vi "Host_HoppingScan(XZ_FPGAWithin).vi"() -> ()   [LabVIEW 2014]
uses:
  <vilib>/userdefined/High Color/nirio_resource_hc.ctl
  <vilib>/Native 3D Graph/xcontrol/3DPC_SurfacePlot.xctl
  <vilib>/Instr/_visa.llb/VISA Configure Serial Port (Instr).vi
  <vilib>/FPGAPlugInAG/PCIe-7851R/niLvFpga_Open_PCIe-7851R.vi
  <vilib>/rvi/interface/common/dynamic/niFpgaDynamicAddResources.vi
  <vilib>/Utility/error.llb/Error Cluster From Error Code.vi
  <vilib>/rvi/errors/niLvFpgaAdjustHostInterfaceError.vi
  <vilib>/FPGAPlugInAG/Dynamic/niLvFpga_Close_Dynamic.vi
  <vilib>/rvi/interface/nirviOpenFPGA/nirviOpenFPGA.xnode
  FPGA Bitfiles/XZFPGAWithinHopp_FPGATarget_HoppingStep(Nonl_ZQj-tD8XJbo.lvbitx
  <vilib>/rvi/interface/nirviReadWriteControl/nirviReadWriteControl.xnode
  <vilib>/rvi/interface/nirviMethod/nirviMethod.xnode
  <vilib>/rvi/interface/nirviCloseFPGA/nirviCloseFPGA.xnode
  NiFpgaLv.dll
  <vilib>/rvi/interface/Simulation/niFpgaSimulationCallBeginRW.vi
  <vilib>/FPGAPlugInAG/Dynamic/niLvFpga_ReadFifo_Dynamic.vi
  <vilib>/rvi/errors/niLvFpgaMergeErrorWithErrorCode.vi
  <vilib>/FPGAPlugInAG/Dynamic/niLvFpga_StopFifo_Dynamic.vi
panel:
  out "XGetNum":u32
  in  "Relative?":bool
  in  "BottomSleep us":i32
  in  "UpperSleep us":i32
  out "SecElapsed s":dbl
  in  "UseCompensation":bool
  in  "Compensation / line":i32
  in  "RelativeWithdraw index":i32
  out "YPresPos":i32
  out "XBuffer":u32
  out "Waveform Chart":i32(graph)
  out "3D Graph":refnum<class "Base Datatype.lvclass">[](xcontrol)
  in  "stop":bool
  in  "ZOffset index":i32
  out "YPos?":dbl
  in  "YNum":i16
  in  "XNum":i16
  in  "YStepLen um":dbl format="%#_13g"
  in  "XStepMultiplier / 0.47nm":i16
  in  "XInitPos um":dbl format="%#_13g"
  in  "YInitPos um":dbl format="%#_13g"
  in  "PIXZ":T1
  out "ERR?":string
  in  "PIYDigital":refnum<visa-resource-name>
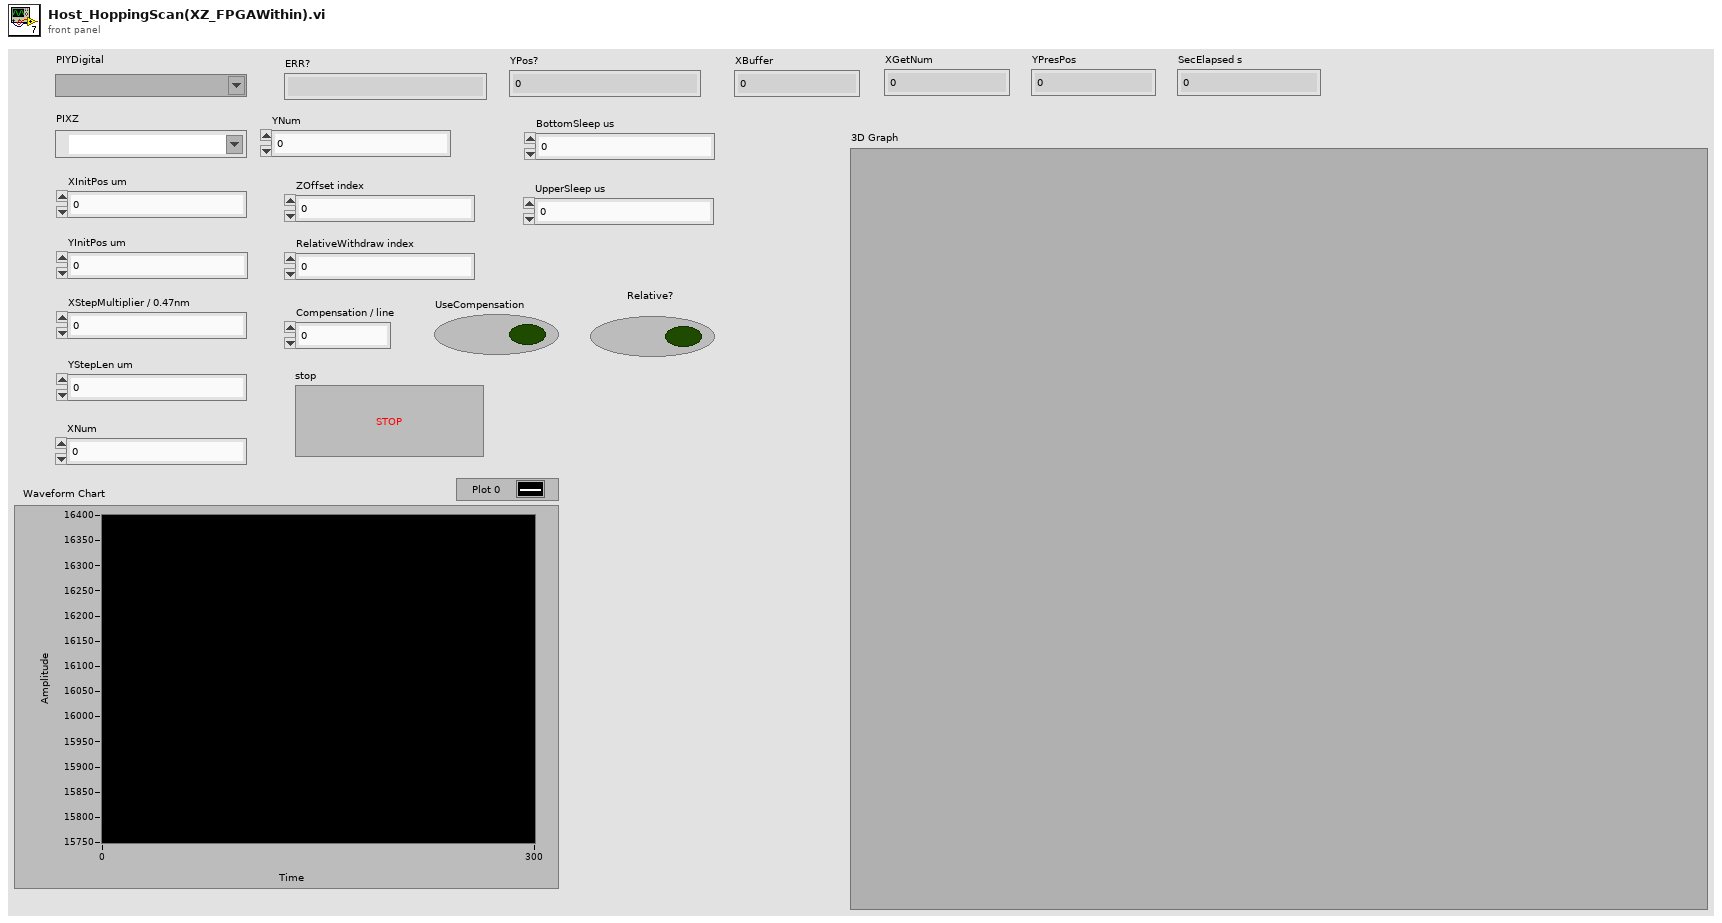
[diagram p1: front panel]
types:
  T1 = typedef "nirio_resource_hc.ctl" = tag
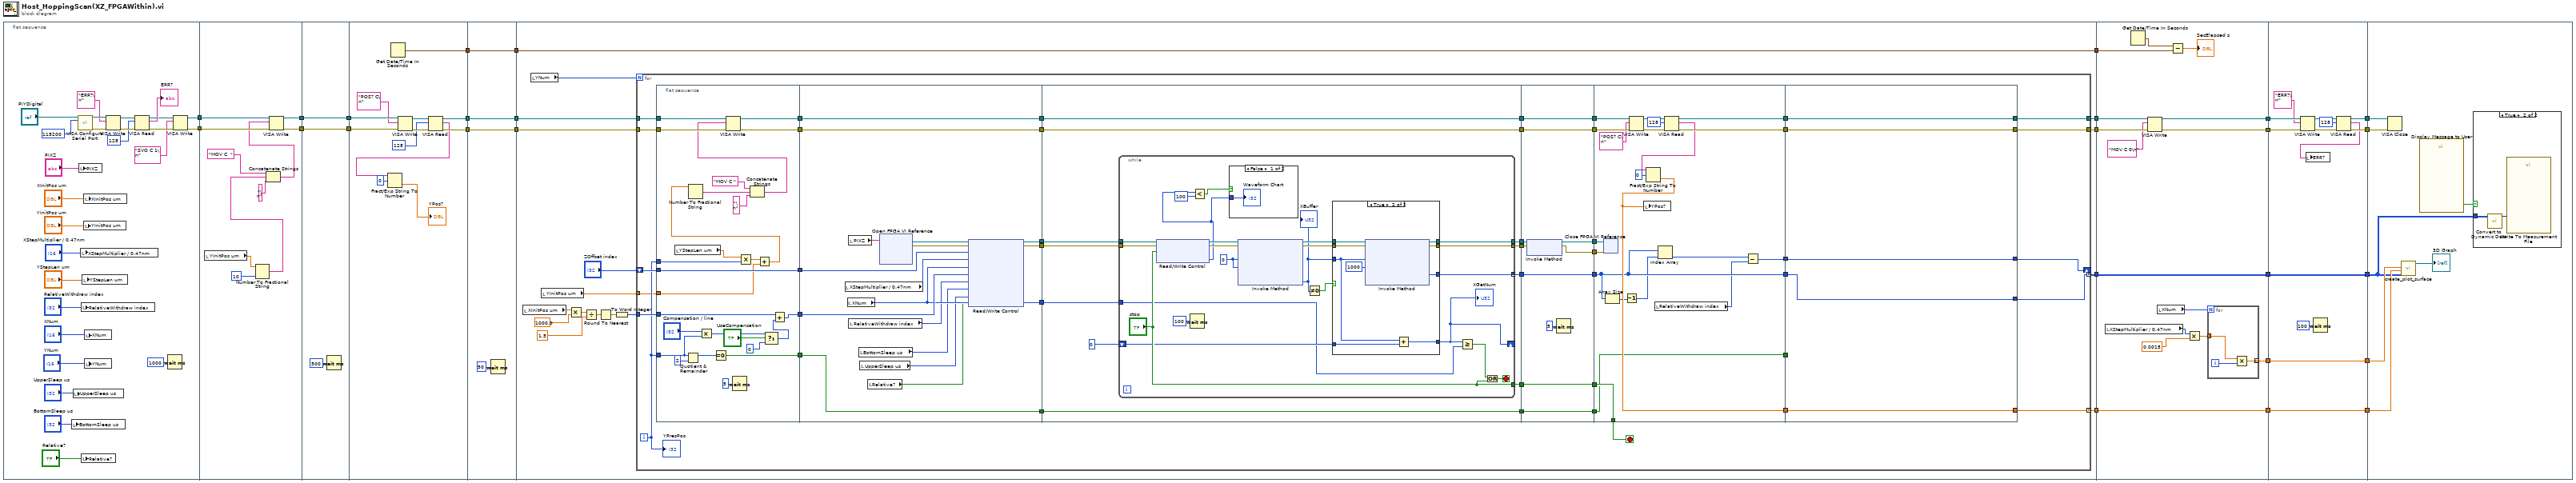
[diagram p0: block diagram]
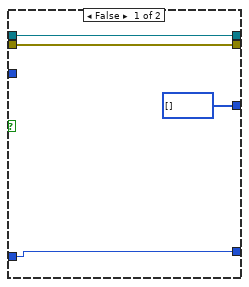
[diagram p3: hidden frame]
diagram:
  n1 = flat-sequence {
    tunnel: [w33] -> w27
    tunnel: [w32] -> w26
    tunnel: w27 -> [w63]
    tunnel: w26 -> [w62]
    tunnel: [w58] -> w25
    tunnel: [w57] -> w24
    tunnel: w25 -> [w65]
    tunnel: w24 -> [w64]
    tunnel: [w65] -> w23
    tunnel: [w64] -> w22
    tunnel: w23 -> [w78]
    tunnel: w22 -> [w77]
    tunnel: [w72] -> w21
    tunnel: [w71] -> w20
    tunnel: [w67] -> w2
    tunnel: w21 -> [w81]
    tunnel: w20 -> [w80]
    tunnel: [w81] -> w19
    tunnel: [w80] -> w18
    tunnel: [w79] -> w3
    tunnel: w2 -> [w79]
    tunnel: w19 -> [w98]
    tunnel: w18 -> [w97]
    tunnel: [w89] -> w17
    tunnel: [w88] -> w16
    tunnel: [w87] -> w11
    tunnel: [w86] -> w10
    tunnel: w3 -> [w83]
    tunnel: [w83] -> w1
    tunnel: w17 -> [w282]
    tunnel: w16 -> [w281]
    tunnel: [w279] -> w15
    tunnel: [w278] -> w14
    tunnel: w11 -> [w271]
    tunnel: w10 -> [w272]
    tunnel: [w273] -> w9
    tunnel: [w272] -> w6
    tunnel: [w271] -> w4
    tunnel: w1 -> [w270]
    tunnel: w15 -> [w298]
    tunnel: w14 -> [w297]
    tunnel: [w292] -> w13
    tunnel: [w291] -> w12
    tunnel: w9 -> [w288]
    tunnel: [w288] -> w8
    tunnel: [w287] -> w7
    tunnel: w6 -> [w287]
    tunnel: [w286] -> w5
    tunnel: w4 -> [w286]
    tunnel: w13 -> [w305]
    tunnel: w12 -> [w304]
    tunnel: w8 -> [w302]
    tunnel: w7 -> [w301]
    tunnel: w5 -> [w299]
    frame #0 {
      n2 = local write "BottomSleep us"("BottomSleep us") -> ()
      n3 = local write "UpperSleep us"("UpperSleep us") -> ()
      n4 = call-poly "VISA Configure Serial Port"("VISA resource name"="PIYDigital", "baud rate (9600)"=u32 115200) -> ("VISA resource name out"=w51:refnum<visa-resource-name>, "error out"=w50:errorcluster)  [unwired: 12 in]
      n5 = local write "PIXZ"("PIXZ") -> ()
      n6 = local write "XStepMultiplier / 0.47nm"("XStepMultiplier / 0.47nm") -> ()
      n7 = local write "RelativeWithdraw index"("RelativeWithdraw index") -> ()
      n8 = local write "Relative?"("Relative?") -> ()
      n9 = local write "YStepLen um"("YStepLen um") -> ()
      n10 = local write "YInitPos um"("YInitPos um") -> ()
      n11 = local write "XInitPos um"("XInitPos um") -> ()
      n12 = local write "XNum"("XNum") -> ()
      n13 = local write "YNum"("YNum") -> ()
      n14 = VISA Write(VISA resource name=w51, write buffer="ERR?\n", error in (no error)=w50) -> (VISA resource name out=w48:refnum<visa-resource-name>, error out=w47:errorcluster)  [unwired: 1 out]
      n15 = VISA Read(VISA resource name=w48, byte count=u32 128, error in (no error)=w47) -> (VISA resource name out=w35:refnum<visa-resource-name>, read buffer=→"ERR?":string, error out=w34:errorcluster)  [unwired: 1 out]
      n16 = Wait (ms)(milliseconds to wait=u32 1000) -> ()  [unwired: 1 out]
      n17 = VISA Write(VISA resource name=w35, write buffer="SVO C 1\n", error in (no error)=w34) -> (VISA resource name out=w33:refnum<visa-resource-name>, error out=w32:errorcluster)  [unwired: 1 out]
    }
    frame #1 {
      n18 = local read "YInitPos um"() -> (w56:dbl)
      n19 = Number To Fractional String(number=w56, precision (6)=i16 10) -> (F-format string=w54:string)  [unwired: 2 in]
      n20 = Concatenate Strings("MOV C  " ("write buffer"), w54, "\n" ("string")) -> (w59:string)
      n21 = VISA Write(VISA resource name=w63, write buffer=w59, error in (no error)=w62) -> (VISA resource name out=w58:refnum<visa-resource-name>, error out=w57:errorcluster)  [unwired: 1 out]
    }
    frame #2 {
      n22 = Wait (ms)(milliseconds to wait=u32 500) -> ()  [unwired: 1 out]
    }
    frame #3 {
      n23 = Get Date/Time In Seconds() -> (seconds since 1Jan1904=w67:timestamp)
      n24 = VISA Write(VISA resource name=w78, write buffer="POS? C\n", error in (no error)=w77) -> (VISA resource name out=w75:refnum<visa-resource-name>, error out=w74:errorcluster)  [unwired: 1 out]
      n25 = VISA Read(VISA resource name=w75, byte count=u32 128, error in (no error)=w74) -> (VISA resource name out=w72:refnum<visa-resource-name>, read buffer=w70:string, error out=w71:errorcluster)  [unwired: 1 out]
      n26 = Fract/Exp String To Number(string=w70, offset=0) -> (number=→"YPos?":dbl)  [unwired: 2 in, 1 out]
    }
    frame #4 {
      n27 = Wait (ms)(milliseconds to wait=u32 50) -> ()  [unwired: 1 out]
    }
    frame #5 {
      n28 = local read "XInitPos um"() -> (w91:dbl)
      n29 = local read "YNum"() -> (w99:i16)
      n30 = local read "YInitPos um"() -> (w84:dbl)
      n31 = Multiply(x=w91, y=1000.0) -> (x*y=w93:dbl)
      n32 = Divide(x=w93, y=1.5) -> (x/y=w95:dbl)
      n33 = Round To Nearest(number=w95) -> (nearest integer value=w96:dbl)
      n34 = To Word Integer(number=w96) -> (16bit integer=w90:i16)
      n35 = for {
        N: w99 -> [_]
        tunnel: w98 -> [w142]
        tunnel: w97 -> [w141]
        tunnel: w90 -> [w135]
        tunnel: [w127] -> w89
        tunnel: [w126] -> w88
        tunnel: [w107] -> w87 mode=indexing
        tunnel: [w118] -> w86 mode=indexing
        shift-right: [w113] -> _
        shift-left: "ZOffset index" -> [w116]
        tunnel: w84 -> [w100]
        i -> [w115]
        stop <- w121 stop-if-true
        n36 = flat-sequence {
          tunnel: w142 -> [w167]
          tunnel: w141 -> [w166]
          tunnel: w115 -> [w168]
          tunnel: [w165] -> w140
          tunnel: [w164] -> w139
          tunnel: [w149] -> w136
          tunnel: w135 -> [w150]
          tunnel: [w158] -> w117
          tunnel: w116 -> [w158]
          tunnel: w115 -> [w147]
          tunnel: [w155] -> w114
          tunnel: w100 -> [w152]
          tunnel: [w181] -> w138
          tunnel: [w180] -> w137
          tunnel: [w176] -> w134
          tunnel: [w175] -> w133
          tunnel: [w177] -> w130
          tunnel: w117 -> [w174]
          tunnel: w136 -> [w178]
          tunnel: w139 -> [w180]
          tunnel: w140 -> [w181]
          tunnel: w114 -> [w173]
          tunnel: [w173] -> w106
          tunnel: w138 -> [w195]
          tunnel: w137 -> [w194]
          tunnel: w134 -> [w187]
          tunnel: w133 -> [w186]
          tunnel: [w195] -> w132
          tunnel: [w194] -> w131
          tunnel: w130 -> [w193]
          tunnel: [w192] -> w129
          tunnel: [w191] -> w128
          tunnel: [w190] -> w123
          tunnel: [w189] -> w119
          tunnel: w106 -> [w188]
          tunnel: [w188] -> w105
          tunnel: w132 -> [w241]
          tunnel: w131 -> [w240]
          tunnel: w129 -> [w236]
          tunnel: w128 -> [w235]
          tunnel: [w241] -> w125
          tunnel: [w240] -> w124
          tunnel: w123 -> [w238]
          tunnel: [w238] -> w122
          tunnel: [w237] -> w120
          tunnel: w119 -> [w237]
          tunnel: w105 -> [w234]
          tunnel: [w234] -> w104
          tunnel: [w233] -> w102
          tunnel: [w232] -> w101
          tunnel: w125 -> [w262]
          tunnel: w124 -> [w261]
          tunnel: w122 -> [w252]
          tunnel: [w252] -> w121
          tunnel: w120 -> [w249]
          tunnel: [w258] -> w112
          tunnel: [w257] -> w111
          tunnel: [w249] -> w110
          tunnel: [w251] -> w109
          tunnel: [w245] -> w108
          tunnel: w104 -> [w244]
          tunnel: [w244] -> w103
          tunnel: w102 -> [w243]
          tunnel: w101 -> [w242]
          tunnel: [w264] -> w113
          tunnel: [w265] -> w118
          tunnel: [w266] -> w126
          tunnel: [w267] -> w127
          tunnel: w112 -> [w267]
          tunnel: w111 -> [w266]
          tunnel: w110 -> [w263]
          tunnel: w109 -> [w265]
          tunnel: w108 -> [w264]
          tunnel: [w263] -> w107
          tunnel: w103 -> [_]
          frame #0 {
            n37 = local read "YStepLen um"() -> (w163:dbl)
            n38 = Quotient & Remainder(x=w147, y=2) -> (x-y*floor(x/y)=w156:i32)  [unwired: 1 out]
            n39 = Multiply(x="Compensation / line", y=w147) -> (x*y=w146:i32)
            n40 = Equal To 0?(x=w156) -> (x = 0?=w155:bool)
            n41 = Wait (ms)(milliseconds to wait=u32 5) -> ()  [unwired: 1 out]
            n42 = Multiply(x=w163, y=w168) -> (x*y=w153:dbl)
            n43 = Add(x=w153, y=w152) -> (x+y=w151:dbl)
            n44 = Number To Fractional String(number=w151) -> (F-format string=w162:string)  [unwired: 3 in]
            n45 = Concatenate Strings("MOV C " ("string"), w162, "\n" ("string")) -> (w159:string)
            n46 = VISA Write(VISA resource name=w167, write buffer=w159, error in (no error)=w166) -> (VISA resource name out=w165:refnum<visa-resource-name>, error out=w164:errorcluster)  [unwired: 1 out]
            n47 = Select(t=w146, s="UseCompensation", f=0) -> (s? t:f=w143:i32)
            n48 = Add(x=w150, y=w143) -> (x+y=w149:i32)
          }
          frame #1 {
            n49 = local read "XStepMultiplier / 0.47nm"() -> (w179:i16)
            n50 = local read "XNum"() -> (w177:i16)
            n51 = local read "PIXZ"() -> (w184:T1)
            n52 = local read "RelativeWithdraw index"() -> (w172:i32)
            n53 = local read "BottomSleep us"() -> (w171:i32)
            n54 = local read "UpperSleep us"() -> (w170:i32)
            n55 = local read "Relative?"() -> (w169:bool)
            n56 = xnode "Open FPGA VI Reference"("resource name"=w184) -> ("FPGA VI Reference Out"=w183:refnum<k20>, "error out"=w182:errorcluster)  [unwired: 1 in]
            n57 = xnode "Read/Write Control"("FPGA VI Reference In"=w183, "error in"=w182, "ZOffset"=w174, "XStepIndex"=w179, "XNum"=w177, "XOffset"=w178, "RelativeWithdraw"=w172, "BottomSleep us"=w171, "UpperSleep us"=w170, "Relative?"=w169) -> ("FPGA VI Reference Out"=w176:refnum<k20>, "error out"=w175:errorcluster)
          }
          frame #2 {
            n58 = while {
              tunnel: w187 -> [w210]
              tunnel: w186 -> [w209]
              tunnel: w193 -> [w197]
              tunnel: [w213] -> w192
              tunnel: [w212] -> w191
              tunnel: ["stop"] -> w190
              tunnel: [w206] -> w189 mode=concatenating
              shift-right: [w196] -> _
              shift-left: 0 -> [w199]
              stop <- w211 stop-if-true
              w216 = u32 0 ("Number of Elements")
              n59 = xnode "Read/Write Control"("FPGA VI Reference In"=w210, "error in"=w209, "stop"="stop") -> ("FPGA VI Reference Out"=w208:refnum<k20>, "error out"=w207:errorcluster, "Waveform Chart"=w202:i32)
              n60 = Wait (ms)(milliseconds to wait=u32 100) -> ()  [unwired: 1 out]
              n61 = Less?(x=w202, y=100) -> (x < y?=w203:bool)
              n62 = case shown="False" w203 {
                tunnel: w202 -> [w218 _]
                frame False {
                  "Waveform Chart" <- w218
                }
                frame True {
                }
              }
              n63 = xnode "Invoke Method"("FPGA VI Reference In"=w208, "error in"=w207, "Number of Elements"=w216, "Timeout (ms)"=w216) -> ("FPGA VI Reference Out"=w215:refnum<k20>, "error out"=w214:errorcluster, "Elements Remaining"=w200:u32)  [unwired: 1 out]
              "XBuffer" <- w200
              n64 = Not Equal To 0?(x=w200) -> (x != 0?=w201:bool)
              n65 = case shown="True" w201 {
                tunnel: w215 -> [w222 w231]
                tunnel: w214 -> [w221 w230]
                tunnel: [w222 w228] -> w213
                tunnel: [w221 w227] -> w212
                tunnel: [i16[] [] ("Data") w226] -> w206
                tunnel: w200 -> [_ w224]
                tunnel: w199 -> [w219 w225]
                tunnel: [w219 w223] -> w196
                frame False {
                }
                frame True {
                  n66 = xnode "Invoke Method"("FPGA VI Reference In"=w231, "error in"=w230, "Number of Elements"=w224, "Timeout (ms)"=1000) -> ("FPGA VI Reference Out"=w228:refnum<k20>, "error out"=w227:errorcluster, "Data"=w226:i16[])  [unwired: 1 out]
                  n67 = Add(x=w224, y=w225) -> (x+y=w223:u32)
                }
              }
              "XGetNum" <- w196
              n68 = Greater Or Equal?(x=w196, y=w197) -> (x >= y?=w198:bool)
              n69 = Or(x=w198, y="stop") -> (x .or. y?=w211:bool)
            }
          }
          frame #3 {
            n70 = xnode "Invoke Method"("FPGA VI Reference In"=w236, "error in"=w235) -> ("FPGA VI Reference Out"=w233:refnum<k20>, "error out"=w232:errorcluster)
            n71 = Wait (ms)(milliseconds to wait=u32 5) -> ()  [unwired: 1 out]
          }
          frame #4 {
            n72 = xnode "Close FPGA VI Reference"("FPGA VI Reference In"=w243, "error in"=w242) -> ()  [unwired: 1 out]
            n73 = Array Size(array=w249) -> (size(s)=w250:i32)
            n74 = Decrement(x=w250) -> (x-1=w248:i32)
            n75 = VISA Write(VISA resource name=w262, write buffer="POS? C\n", error in (no error)=w261) -> (VISA resource name out=w260:refnum<visa-resource-name>, error out=w259:errorcluster)  [unwired: 1 out]
            n76 = local read "RelativeWithdraw index"() -> (w246:i32)
            n77 = Index Array(array=w249, index=w248) -> (element=w247:i16)
            n78 = VISA Read(VISA resource name=w260, byte count=u32 128, error in (no error)=w259) -> (VISA resource name out=w258:refnum<visa-resource-name>, read buffer=w254:string, error out=w257:errorcluster)  [unwired: 1 out]
            n79 = Fract/Exp String To Number(string=w254, offset=0) -> (number=w251:dbl)  [unwired: 2 in, 1 out]
            n80 = local write "YPos?"(w251) -> ()
            n81 = Subtract(x=w247, y=w246) -> (x-y=w245:i32)
          }
          frame #5 {
          }
        }
        "YPresPos" <- w115
      }
    }
    frame #6 {
      n82 = local read "XStepMultiplier / 0.47nm"() -> (w276:i16)
      n83 = Get Date/Time In Seconds() -> (seconds since 1Jan1904=w269:timestamp)
      n84 = VISA Write(VISA resource name=w282, write buffer="MOV C 0\n", error in (no error)=w281) -> (VISA resource name out=w279:refnum<visa-resource-name>, error out=w278:errorcluster)  [unwired: 1 out]
      n85 = local read "XNum"() -> (w277:i16)
      n86 = Subtract(x=w269, y=w270) -> (x-y=→"SecElapsed s":dbl)
      n87 = Multiply(x=w276, y=0.0015) -> (x*y=w274:dbl)
      n88 = for {
        N: w277 -> [_]
        tunnel: w274 -> [w285]
        tunnel: [w283] -> w273 mode=indexing
        i -> [w284]
        n89 = Multiply(x=w285, y=w284) -> (x*y=w283:dbl)
      }
    }
    frame #7 {
      n90 = VISA Write(VISA resource name=w298, write buffer="ERR?\n", error in (no error)=w297) -> (VISA resource name out=w295:refnum<visa-resource-name>, error out=w294:errorcluster)  [unwired: 1 out]
      n91 = Wait (ms)(milliseconds to wait=u32 100) -> ()  [unwired: 1 out]
      n92 = VISA Read(VISA resource name=w295, byte count=u32 128, error in (no error)=w294) -> (VISA resource name out=w292:refnum<visa-resource-name>, read buffer=w290:string, error out=w291:errorcluster)  [unwired: 1 out]
      n93 = local write "ERR?"(w290) -> ()
    }
    frame #8 {
      n94 = VISA Close(VISA resource name=w305, error in (no error)=w304) -> ()  [unwired: 1 out]
      n95 = call <vilib>:"create_plot_surface.vi"("z matrix"=w299, "y vector"=w301, "x vector"=w302) -> ("plots out"=→"3D Graph":refnum<class "Base Datatype.lvclass">[])  [unwired: 2 in, 6 out]
      n96 = call "Display Message to User"() -> ("OK"=w300:bool)  [unwired: 10 in, 1 out]
      n97 = case shown="True" w300 {
        tunnel: w299 -> [_ w307]
        frame False {
        }
        frame True {
          n98 = call "Convert to Dynamic Data"("2D Array"=w307) -> ("Dynamic Data Type"=w306:dynamicdata)  [unwired: 3 in]
          n99 = call "Write To Measurement File"("Signals"=w306) -> ()  [unwired: 16 in, 3 out]
        }
      }
    }
  }
